vi "Read Calibration Data Array.vi"(5 "Port (1)":i32=1, 7 "Channel (1)":i32=1, 8 "error in (no error)":errorcluster, 11 "VISA resource name":refnum<visa-resource-name>) -> (0 "error out":errorcluster, 2 "Calibration Data Array":dbl[](array[numeric]), 3 "VISA resource name out":refnum<visa-resource-name>)   [LabVIEW 2011, in "Agilent ENA Series.lvlib"]
doc: "For selected port of selected channel, reads out the power calibration data array."
uses:
  Agilent ENA Series.lvlib
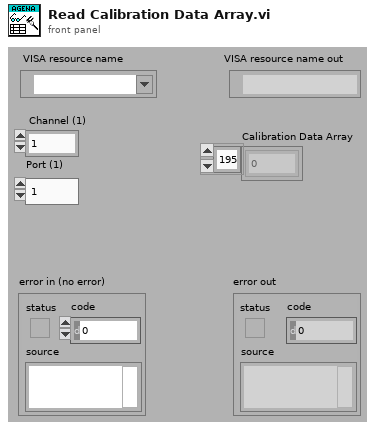
[diagram p1: front panel]
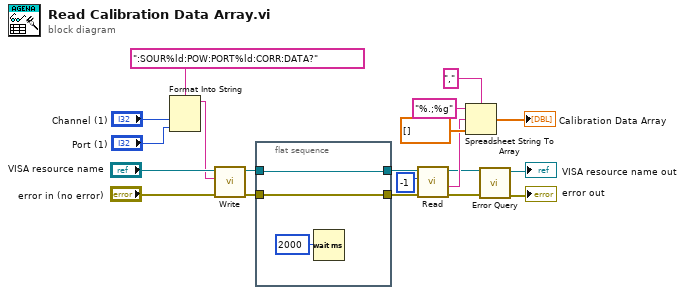
[diagram p0: block diagram]
diagram:
  n1 = Format Into String(format string=":SOUR%ld:POW:PORT%ld:CORR:DATA?", "Channel (1)", "Port (1)") -> (resulting string=w16:string)  [unwired: 2 in, 1 out]
  n2 = call "Write.vi"("error in (no error)"="error in (no error)", "String ()"=w16, "VISA resource name"="VISA resource name") -> ("error out"=w8:errorcluster, "VISA resource name out"=w9:refnum<visa-resource-name>)  [unwired: 6 in, 1 out]
  n3 = flat-sequence {
    tunnel: w9 -> [w22]
    tunnel: w8 -> [w21]
    tunnel: [w22] -> w6
    tunnel: [w21] -> w7
    frame #0 {
      n4 = Wait (ms)(milliseconds to wait=2000) -> ()  [unwired: 1 out]
    }
  }
  n5 = call "Read.vi"("error in (no error)"=w7, "Number Of Bytes"=-1, "VISA resource name"=w6) -> ("error out"=w3:errorcluster, "String"=w5:string, "VISA resource name out"=w4:refnum<visa-resource-name>)  [unwired: 5 in, 1 out]
  n6 = Spreadsheet String To Array(delimiter (Tab)=",", format string="%.;%g", spreadsheet string=w5, array type (2D Dbl)=dbl[] []) -> (array=→"Calibration Data Array":dbl[])
  n7 = call "Error Query.vi"("error in (no error)"=w3, "VISA resource name"=w4) -> ("error out"=→"error out":errorcluster, "VISA resource name out"=→"VISA resource name out":refnum<visa-resource-name>)  [unwired: 6 in, 2 out]
